vi "If Else Y.vi"(0 "denge degeri":dbl, 5 "Yk":dbl, 7 "Y(k-1)":dbl=0.1, 9 "output y 1":dbl, 11 "output y 2":dbl, 12 "result output y":dbl) -> (4 "Output Y(k-1)":dbl format="%.4p", 15 "Start Y":bool)   [LabVIEW 2014]
uses:
  Sub_VI/show_sensitivity.vi
  Sub_VI/global get findinput.vi
panel:
  out "cycle":bool
  in  "GPIB In":refnum<visa-resource-name>="GPIB0::8::INSTR"
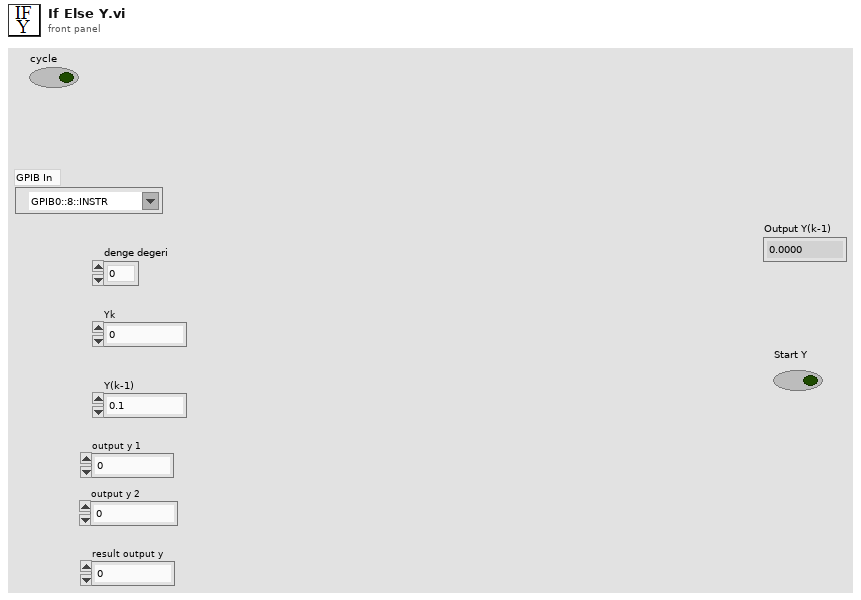
[diagram p1: front panel]
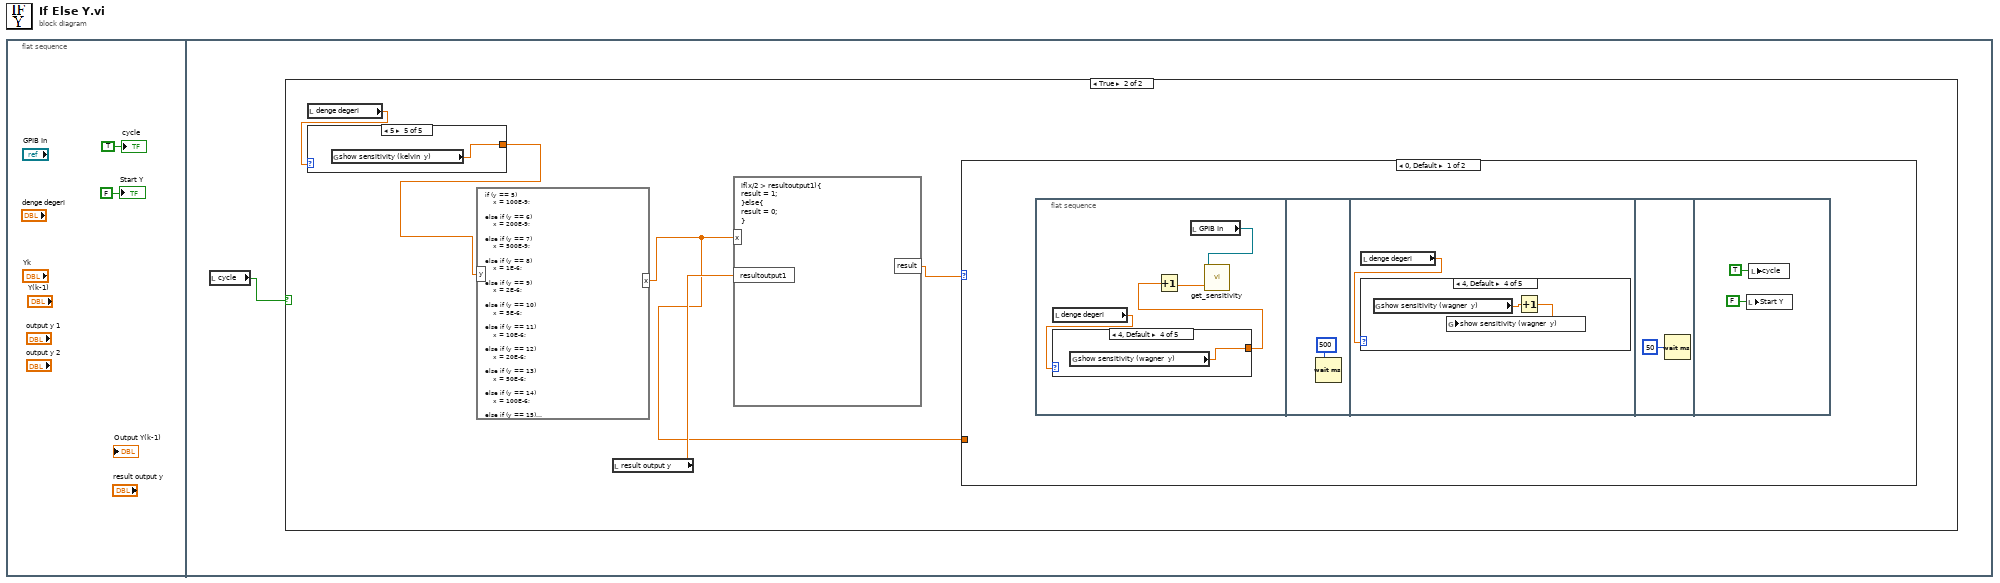
[diagram p0: block diagram]
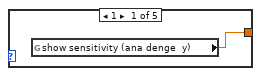
[diagram p3: hidden frame]
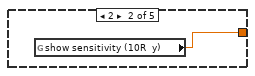
[diagram p4: hidden frame]
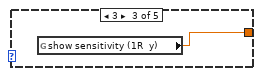
[diagram p5: hidden frame]
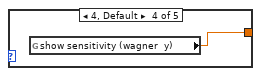
[diagram p6: hidden frame]
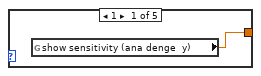
[diagram p7: hidden frame]
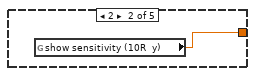
[diagram p8: hidden frame]
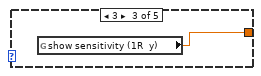
[diagram p9: hidden frame]
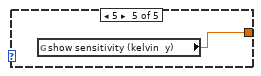
[diagram p10: hidden frame]
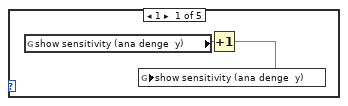
[diagram p11: hidden frame]
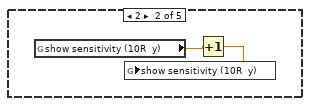
[diagram p12: hidden frame]
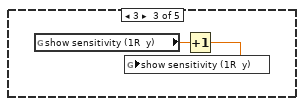
[diagram p13: hidden frame]
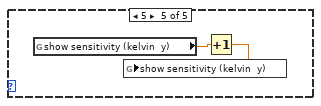
[diagram p14: hidden frame]
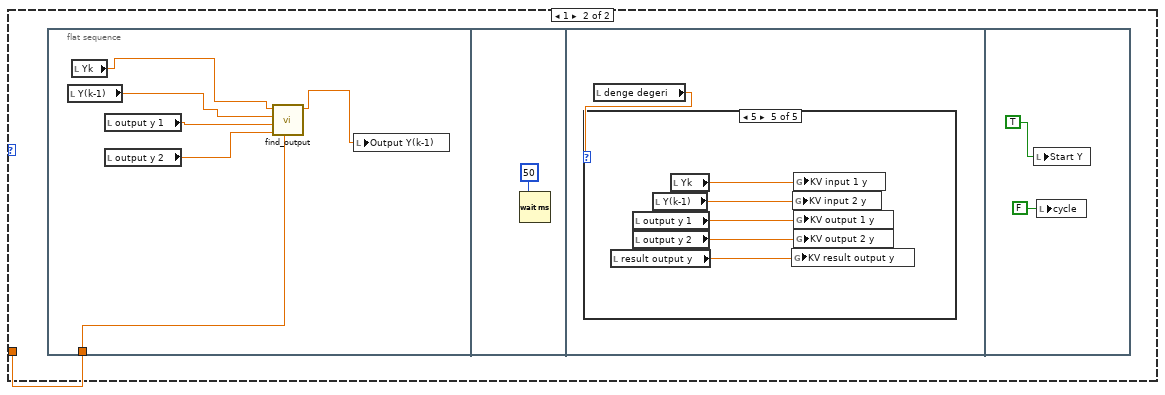
[diagram p15: hidden frame]
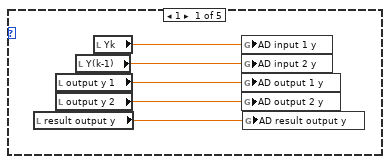
[diagram p16: hidden frame]
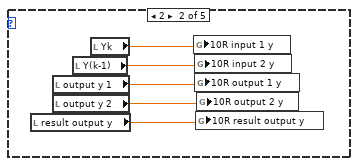
[diagram p17: hidden frame]
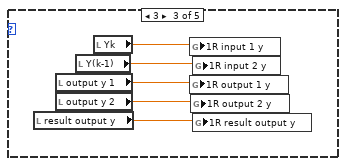
[diagram p18: hidden frame]
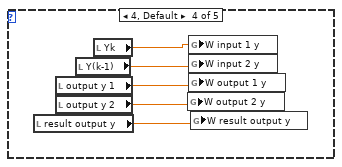
[diagram p19: hidden frame]
diagram:
  n1 = flat-sequence {
    frame #0 {
      "Start Y" <- FALSE ("Start Y")
      "cycle" <- TRUE ("cycle")
    }
    frame #1 {
      n2 = local read "cycle"() -> (w3:bool)
      n3 = case shown="True" w3 {
        frame False {
        }
        frame True {
          n4 = local read "denge degeri"() -> (w5:dbl)
          n5 = case shown="5" w5 {
            tunnel: [w9 w10 w11 w12 w13] -> w4
            frame 1 {
              n6 = global read "show_sensitivity.vi" "show sensitivity (ana denge  y)"() -> (w9:dbl)
            }
            frame 2 {
              n7 = global read "show_sensitivity.vi" "show sensitivity (10R  y)"() -> (w10:dbl)
            }
            frame 3 {
              n8 = global read "show_sensitivity.vi" "show sensitivity (1R  y)"() -> (w11:dbl)
            }
            frame 4, Default {
              n9 = global read "show_sensitivity.vi" "show sensitivity (wagner  y)"() -> (w12:dbl)
            }
            frame 5 {
              n10 = global read "show_sensitivity.vi" "show sensitivity (kelvin  y)"() -> (w13:dbl)
            }
          }
          n11 = formula code="if (y == 5) \n    x = 100E-9;\n\nelse if (y == 6) \n    x = 200E-9;\n\nelse if (y == 7) \n    x = 500E-9;\n\nelse if (y == 8) \n    x = 1E-6;\n\nelse if (y == 9) \n    x = 2E-6;\n\nelse if (y == 10) \n    x = 5E-6;\n\nelse if (y == 11) \n    x = 10E-6;\n\nelse if (y == 12) \n    x = 20E-6;\n\nelse if (y == 13) \n    x = 50E-6;\n\nelse if (y == 14) \n    x = 100E-6;\n\nelse if (y == 15) \n    x = 200E-6;\n\nelse if (y == 16) \n    x = 500E-6;\n\nelse if (y == 17) \n    x = 1E-3;\n\nelse if (y == 18) \n    x = 2E-3;\n\nelse if (y == 19) \n    x = 5E-3;\n\nelse if (y == 20) \n    x = 10E-3;\n\nelse if (y == 21) \n    x = 20E-3;\n\nelse if (y == 22) \n    x = 50E-3;\n\nelse if (y == 23) \n    x = 100E-3;\n\nelse if (y == 24) \n    x = 200E-3;\n\nelse if (y == 25) \n    x = 500E-3;\n\nelse if (y == 26) \n    x = 1;\n\nelse \n    x = 1;"("y"=w4) -> ("x"=w6:dbl)
          n12 = local read "result output y"() -> (w8:dbl)
          n13 = formula code="if(x/2 > resultoutput1){\nresult = 1;\n}else{\nresult = 0;\n}"("x"=w6, "resultoutput1"=w8) -> ("result"=w7:dbl)
          n14 = case shown="0, Default" w7 {
            tunnel: w6 -> [_ w38]
            frame 0, Default {
              n15 = flat-sequence {
                frame #0 {
                  n16 = local read "denge degeri"() -> (w15:dbl)
                  n17 = case shown="4, Default" w15 {
                    tunnel: [w18 w19 w20 w21 w22] -> w14
                    frame 1 {
                      n18 = global read "show_sensitivity.vi" "show sensitivity (ana denge  y)"() -> (w18:dbl)
                    }
                    frame 2 {
                      n19 = global read "show_sensitivity.vi" "show sensitivity (10R  y)"() -> (w19:dbl)
                    }
                    frame 3 {
                      n20 = global read "show_sensitivity.vi" "show sensitivity (1R  y)"() -> (w20:dbl)
                    }
                    frame 4, Default {
                      n21 = global read "show_sensitivity.vi" "show sensitivity (wagner  y)"() -> (w21:dbl)
                    }
                    frame 5 {
                      n22 = global read "show_sensitivity.vi" "show sensitivity (kelvin  y)"() -> (w22:dbl)
                    }
                  }
                  n23 = Increment(x=w14) -> (x+1=w16:dbl)
                  n24 = local read "GPIB In"() -> (w17:refnum<visa-resource-name>)
                  n25 = call "get_sensitivity.vi"("input 1"=w16, "SR850 GPIB In"=w17) -> ()  [unwired: 8 in, 2 out]
                }
                frame #1 {
                  n26 = Wait (ms)(milliseconds to wait=u32 500) -> ()  [unwired: 1 out]
                }
                frame #2 {
                  n27 = local read "denge degeri"() -> (w24:dbl)
                  n28 = case shown="4, Default" w24 {
                    frame 1 {
                      n29 = global read "show_sensitivity.vi" "show sensitivity (ana denge  y)"() -> (w26:dbl)
                      n30 = Increment(x=w26) -> (x+1=w25:dbl)
                      n31 = global write "show_sensitivity.vi" "show sensitivity (ana denge  y)"(w25) -> ()
                    }
                    frame 2 {
                      n32 = global read "show_sensitivity.vi" "show sensitivity (10R  y)"() -> (w28:dbl)
                      n33 = Increment(x=w28) -> (x+1=w27:dbl)
                      n34 = global write "show_sensitivity.vi" "show sensitivity (10R  y)"(w27) -> ()
                    }
                    frame 3 {
                      n35 = global read "show_sensitivity.vi" "show sensitivity (1R  y)"() -> (w30:dbl)
                      n36 = Increment(x=w30) -> (x+1=w29:dbl)
                      n37 = global write "show_sensitivity.vi" "show sensitivity (1R  y)"(w29) -> ()
                    }
                    frame 4, Default {
                      n38 = global read "show_sensitivity.vi" "show sensitivity (wagner  y)"() -> (w32:dbl)
                      n39 = Increment(x=w32) -> (x+1=w31:dbl)
                      n40 = global write "show_sensitivity.vi" "show sensitivity (wagner  y)"(w31) -> ()
                    }
                    frame 5 {
                      n41 = global read "show_sensitivity.vi" "show sensitivity (kelvin  y)"() -> (w34:dbl)
                      n42 = Increment(x=w34) -> (x+1=w33:dbl)
                      n43 = global write "show_sensitivity.vi" "show sensitivity (kelvin  y)"(w33) -> ()
                    }
                  }
                }
                frame #3 {
                  n44 = Wait (ms)(milliseconds to wait=u32 50) -> ()  [unwired: 1 out]
                }
                frame #4 {
                  n45 = local write "Start Y"(FALSE ("Start X")) -> ()
                  n46 = local write "cycle"(TRUE ("cycle")) -> ()
                }
              }
            }
            frame 1 {
              n47 = flat-sequence {
                tunnel: w38 -> [w42]
                frame #0 {
                  n48 = local read "Y(k-1)"() -> (w41:dbl)
                  n49 = local read "Yk"() -> (w40:dbl)
                  n50 = local read "output y 1"() -> (w44:dbl)
                  n51 = local read "output y 2"() -> (w43:dbl)
                  n52 = call "find_output.vi"("find output"=w42, "output 2"=w43, "output 1"=w44, "input 2"=w41, "input 1"=w40) -> ("getInput"=w39:dbl)  [unwired: 6 in]
                  n53 = local write "Output Y(k-1)"(w39) -> ()
                }
                frame #1 {
                  n54 = Wait (ms)(milliseconds to wait=u32 50) -> ()  [unwired: 1 out]
                }
                frame #2 {
                  n55 = local read "denge degeri"() -> (w46:dbl)
                  n56 = case shown="5" w46 {
                    frame 1 {
                      n57 = local read "result output y"() -> (w47:dbl)
                      n58 = local read "output y 1"() -> (w49:dbl)
                      n59 = local read "output y 2"() -> (w48:dbl)
                      n60 = local read "Y(k-1)"() -> (w50:dbl)
                      n61 = local read "Yk"() -> (w51:dbl)
                      n62 = global write "global get findinput.vi" "AD input 1 y"(w51) -> ()
                      n63 = global write "global get findinput.vi" "AD input 2 y"(w50) -> ()
                      n64 = global write "global get findinput.vi" "AD output 1 y"(w49) -> ()
                      n65 = global write "global get findinput.vi" "AD output 2 y"(w48) -> ()
                      n66 = global write "global get findinput.vi" "AD result output y"(w47) -> ()
                    }
                    frame 2 {
                      n67 = local read "result output y"() -> (w52:dbl)
                      n68 = local read "output y 1"() -> (w54:dbl)
                      n69 = local read "output y 2"() -> (w53:dbl)
                      n70 = local read "Y(k-1)"() -> (w55:dbl)
                      n71 = local read "Yk"() -> (w56:dbl)
                      n72 = global write "global get findinput.vi" "10R input 1 y"(w56) -> ()
                      n73 = global write "global get findinput.vi" "10R input 2 y"(w55) -> ()
                      n74 = global write "global get findinput.vi" "10R output 1 y"(w54) -> ()
                      n75 = global write "global get findinput.vi" "10R result output y"(w52) -> ()
                      n76 = global write "global get findinput.vi" "10R output 2 y"(w53) -> ()
                    }
                    frame 3 {
                      n77 = local read "result output y"() -> (w57:dbl)
                      n78 = local read "output y 1"() -> (w59:dbl)
                      n79 = local read "output y 2"() -> (w58:dbl)
                      n80 = local read "Y(k-1)"() -> (w60:dbl)
                      n81 = local read "Yk"() -> (w61:dbl)
                      n82 = global write "global get findinput.vi" "1R input 1 y"(w61) -> ()
                      n83 = global write "global get findinput.vi" "1R output 1 y"(w59) -> ()
                      n84 = global write "global get findinput.vi" "1R output 2 y"(w58) -> ()
                      n85 = global write "global get findinput.vi" "1R input 2 y"(w60) -> ()
                      n86 = global write "global get findinput.vi" "1R result output y"(w57) -> ()
                    }
                    frame 4, Default {
                      n87 = local read "result output y"() -> (w62:dbl)
                      n88 = local read "output y 1"() -> (w64:dbl)
                      n89 = local read "output y 2"() -> (w63:dbl)
                      n90 = local read "Y(k-1)"() -> (w65:dbl)
                      n91 = local read "Yk"() -> (w66:dbl)
                      n92 = global write "global get findinput.vi" "W output 2 y"(w63) -> ()
                      n93 = global write "global get findinput.vi" "W input 1 y"(w66) -> ()
                      n94 = global write "global get findinput.vi" "W input 2 y"(w65) -> ()
                      n95 = global write "global get findinput.vi" "W output 1 y"(w64) -> ()
                      n96 = global write "global get findinput.vi" "W result output y"(w62) -> ()
                    }
                    frame 5 {
                      n97 = local read "result output y"() -> (w67:dbl)
                      n98 = local read "output y 1"() -> (w69:dbl)
                      n99 = local read "output y 2"() -> (w68:dbl)
                      n100 = local read "Y(k-1)"() -> (w70:dbl)
                      n101 = local read "Yk"() -> (w71:dbl)
                      n102 = global write "global get findinput.vi" "KV result output y"(w67) -> ()
                      n103 = global write "global get findinput.vi" "KV input 2 y"(w70) -> ()
                      n104 = global write "global get findinput.vi" "KV input 1 y"(w71) -> ()
                      n105 = global write "global get findinput.vi" "KV output 1 y"(w69) -> ()
                      n106 = global write "global get findinput.vi" "KV output 2 y"(w68) -> ()
                    }
                  }
                }
                frame #3 {
                  n107 = local write "Start Y"(TRUE ("START X")) -> ()
                  n108 = local write "cycle"(FALSE ("cycle")) -> ()
                }
              }
            }
          }
        }
      }
    }
  }
